vi "CanOpen Öffnen.vi"(8 "error in (no error)":errorcluster) -> (0 "Fehler (Ausgang)":errorcluster, 3 "CanOpen Obj":T1={"node-ID"=1, "RPDO1 controlword"=refnum, "TPDO1 status"=refnum, "RPDO2 I-Sollwert"=refnum, "TPDO2 Ist-Werte"=refnum, "SYNC object"=refnum})   [LabVIEW 2014]
uses:
  <vilib>/CANopenLib/CANOPEN.llb/CANopen BaudRate.ctl
  <vilib>/CANopenLib/CANOPEN.llb/CANopen Interface Create.vi
  <vilib>/CANopenLib/CANOPEN.llb/CANopen SYNC Create.vi
  <vilib>/CANopenLib/CANOPEN.llb/CANopen SYNC Start.vi
  <vilib>/CANopenLib/CANOPEN.llb/CANopen TPDO Create.vi
  <vilib>/CANopenLib/CANOPEN.llb/CANopen TPDO Start.vi
  <vilib>/CANopenLib/CANOPEN.llb/CANopen RPDO Create.vi
  <vilib>/CANopenLib/CANOPEN.llb/CANopen RPDO Start.vi
panel:
  in  "node-ID":u8=3
  in  "baud rate":T2 items=["1 Mbit/s"=0, "800 kbit/s"=1, "500 kbit/s"=2, "250 kbit/s"=3, "125 kbit/s"=4, "50 kbit/s"=6, "20 kbit/s"=7, "10 kbit/s"=8]
  in  "interface name":u32(ring) items=["CANopen01", "CANopen02", "CANopen03", "CANopen04", "CANopen05", "CANopen06", "CANopen07", "CANopen08", "CANopen09", "CANopen10", "CANopen11", "CANopen12", "CANopen13", "CANopen14", "CANopen15", "CANopen16", "CANopen17", "CANopen18", "CANopen19", "CANopen20", "CANopen21", "CANopen22", "CANopen23", "CANopen24", "CANopen25", "CANopen26", "CANopen27", "CANopen28", "CANopen29", "CANopen30", "CANopen31", "CANopen32"]
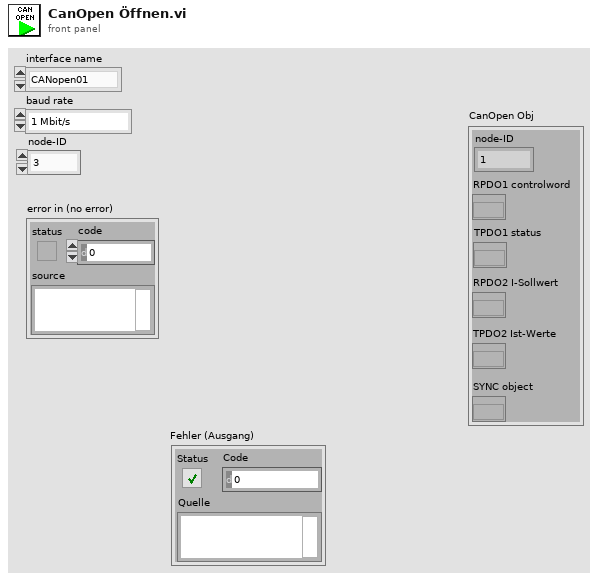
[diagram p1: front panel]
types:
  T1 = cluster{"node-ID":u8, "RPDO1 controlword":refnum<k20>, "TPDO1 status":refnum<k20>, "RPDO2 I-Sollwert":refnum<k20>, "TPDO2 Ist-Werte":refnum<k20>, "SYNC object":refnum<k20>}
  T2 = typedef "CANopen BaudRate.ctl" = u32
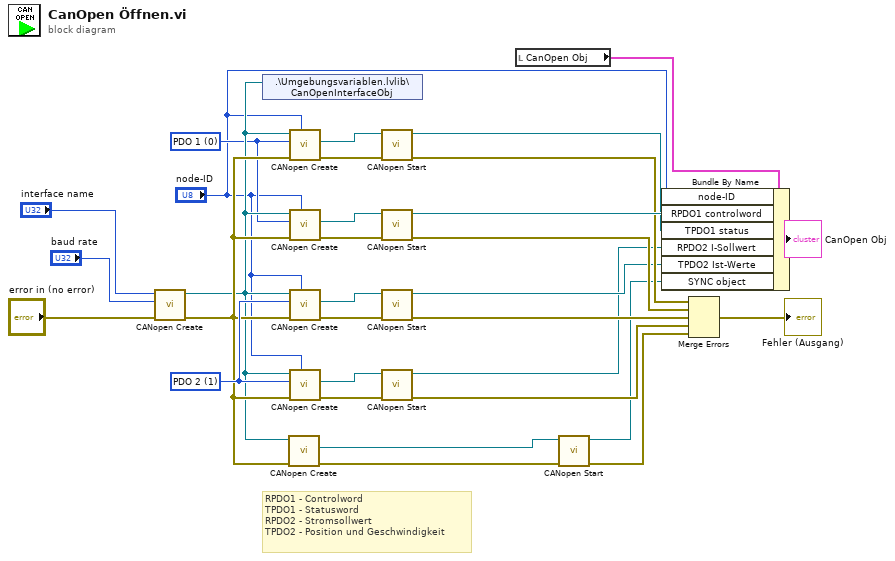
[diagram p0: block diagram]
diagram:
  w12 = u8 1 items=["PDO 1", "PDO 2", "PDO 3", "PDO 4"] ("PDO channel")
  w5 = u8 0 items=["PDO 1", "PDO 2", "PDO 3", "PDO 4"] ("PDO channel")
  # "RPDO1 - Controlword\nTPDO1 - Statusword\nRPDO2 - Stromsollwert\nTPDO2 - Position und Geschwindigkeit"
  n1 = call-poly <vilib>:"CANopen Create.vi"("error in (no error)"="error in (no error)", "baud rate"="baud rate", "interface name"="interface name") -> ("error out"=w11:errorcluster, "interface object out"=w10:refnum<k20>)  [unwired: 7 in]
  n2 = shared-variable ".\\Umgebungsvariablen.lvlib\\CanOpenInterfaceObj"(w10) -> ()  [unwired: 1 in, 1 out]
  n3 = call-poly <vilib>:"CANopen Create.vi"("error in (no error)"=w11, "interface object in"=w10) -> ("error out"=w24:errorcluster, "SYNC object out"=w27:refnum<k20>)  [unwired: 7 in, 1 out]
  n4 = call-poly <vilib>:"CANopen Create.vi"("node-ID"="node-ID", "error in (no error)"=w11, "PDO channel"=w5, "interface object in"=w10) -> ("error out"=w25:errorcluster, "TPDO object out"=w28:refnum<k20>)  [unwired: 5 in, 1 out]
  n5 = call-poly <vilib>:"CANopen Create.vi"("node-ID"="node-ID", "error in (no error)"=w11, "PDO channel"=w5, "interface object in"=w10) -> ("error out"=w26:errorcluster, "RPDO object out"=w29:refnum<k20>)  [unwired: 5 in, 1 out]
  n6 = call-poly <vilib>:"CANopen Create.vi"("node-ID"="node-ID", "error in (no error)"=w11, "PDO channel"=w12, "interface object in"=w10) -> ("error out"=w16:errorcluster, "TPDO object out"=w13:refnum<k20>)  [unwired: 5 in, 1 out]
  n7 = call-poly <vilib>:"CANopen Create.vi"("node-ID"="node-ID", "error in (no error)"=w11, "PDO channel"=w12, "interface object in"=w10) -> ("error out"=w15:errorcluster, "RPDO object out"=w14:refnum<k20>)  [unwired: 5 in, 1 out]
  n8 = call-poly <vilib>:"CANopen Start.vi"("error in (no error)"=w25, "TPDO object in"=w28) -> ("error out"=w7:errorcluster, "TPDO object out"=w19:refnum<k20>)  [unwired: 8 in]
  n9 = call-poly <vilib>:"CANopen Start.vi"("error in (no error)"=w26, "RPDO object in"=w29) -> ("error out"=w23:errorcluster, "RPDO object out"=w20:refnum<k20>)  [unwired: 8 in]
  n10 = call-poly <vilib>:"CANopen Start.vi"("error in (no error)"=w16, "TPDO object in"=w13) -> ("error out"=w9:errorcluster, "TPDO object out"=w2:refnum<k20>)  [unwired: 8 in]
  n11 = call-poly <vilib>:"CANopen Start.vi"("error in (no error)"=w15, "RPDO object in"=w14) -> ("error out"=w8:errorcluster, "RPDO object out"=w1:refnum<k20>)  [unwired: 8 in]
  n12 = local read "CanOpen Obj"() -> (w21:T1)
  n13 = call-poly <vilib>:"CANopen Start.vi"("error in (no error)"=w24, "SYNC object in"=w27) -> ("error out"=w6:errorcluster, "SYNC object out"=w3:refnum<k20>)  [unwired: 8 in]
  n14 = Bundle By Name(cluster=w21, "node-ID"="node-ID", "RPDO1 controlword"=w20, "TPDO1 status"=w19, "RPDO2 I-Sollwert"=w1, "TPDO2 Ist-Werte"=w2, "SYNC object"=w3) -> (→"CanOpen Obj":T1)
  n15 = Merge Errors(w7, w23, w9, w8, w6) -> (→"Fehler (Ausgang)":errorcluster)
